vi "Create Recorder Status Cluster.vi"(8 "error in (no error)":errorcluster, 10 "Frames Written this iteration":i32, 11 "File Reference In":refnum<file>) -> (0 "error out":errorcluster, 2 "Data Recorder Status":T1, 3 "File Reference Out":refnum<file>)   [LabVIEW 2021]
uses:
  Type Definitions/Telemetry Recorder Status.ctl
  <vilib>/ptbypt/NI_PtbyPt.lvlib
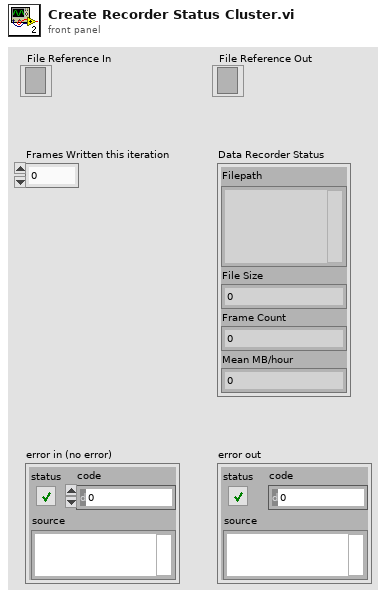
[diagram p1: front panel]
types:
  T1 = typedef "Telemetry Recorder Status.ctl" = cluster{"Filepath":string, "File Size":i64, "Frame Count":i32, "Mean MB/hour":sgl}
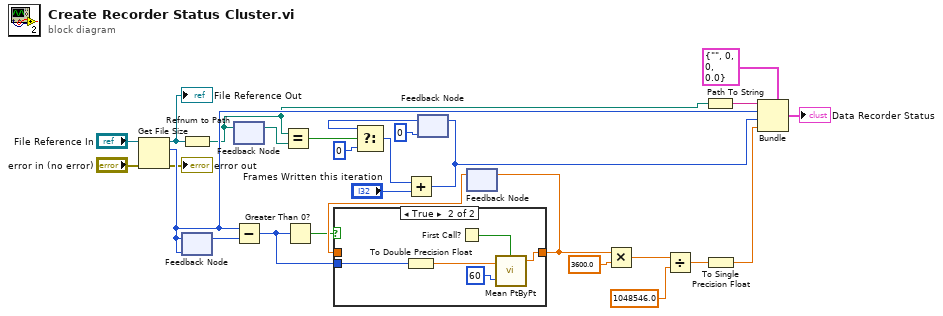
[diagram p0: block diagram]
diagram:
  n1 = Get File Size(file="File Reference In", error in="error in (no error)") -> (refnum out=w1:refnum<file>, size (in bytes)=w18:i64, 0:→"error out":errorcluster)
  "File Reference Out" <- w1
  n2 = Refnum to Path(1:w1) -> (0:w4:path)
  n3 = feedback #1(w18) -> (w15:i64)
  n4 = feedback-in #1(w18) -> ()
  n5 = feedback #2() -> (w5:path)  [unwired: 1 in]
  n6 = feedback-in #2(w4) -> ()
  n7 = Subtract(x=w18, y=w15) -> (x-y=w22:i64)
  n8 = Equal?(x=w4, y=w5) -> (x = y?=w6:bool)
  n9 = Greater Than 0?(x=w22) -> (x > 0?=w23:bool)
  n10 = feedback #3(0) -> (w8:i32)
  n11 = Select(t=w8, s=w6, f=0) -> (s? t:f=w9:i32)
  n12 = Add(x=w9, y="Frames Written this iteration") -> (x+y=w12:i32)
  n13 = feedback-in #3(w12) -> ()
  n14 = feedback #4() -> (w25:dbl)  [unwired: 1 in]
  n15 = case shown="True" w23 {
    tunnel: [w28 w32] -> w24
    tunnel: w22 -> [_ w31]
    tunnel: w25 -> [w28 _]
    frame False {
    }
    frame True {
      n16 = To Double Precision Float(number=w31) -> (double precision float=w30:dbl)
      n17 = First Call?() -> (First Call?: T/F=w29:bool)
      n18 = call <vilib>:"Mean PtByPt.vi"("x"=w30, "sample length"=60, "initialize"=w29) -> ("mean"=w32:dbl)  [unwired: 1 in, 1 out]
    }
  }
  n19 = feedback-in #4(w24) -> ()
  n20 = Multiply(x=w24, y=3600.0) -> (x*y=w19:dbl)
  n21 = Divide(x=w19, y=1048546.0) -> (x/y=w21:dbl)
  n22 = Path To String(path=w4) -> (string=w3:string)
  n23 = To Single Precision Float(number=w21) -> (single precision float=w17:sgl)
  n24 = Bundle(cluster=T1 {"Filepath"="", "File Size"=0, "Frame Count"=0, "Mean MB/hour"=0.0}, "Filepath"=w3, "File Size"=w18, "Frame Count"=w12, "Mean MB/hour"=w17) -> (→"Data Recorder Status":T1)
